vi "Configure.vi"(8 "error in (no error)":errorcluster, 11 "Tomo in":refnum<class "Tomo.lvclass">) -> (0 "error out":errorcluster, 2 "cancelled?":bool, 3 "Tomo out":refnum<class "Tomo.lvclass">)   [LabVIEW 2012, in "Tomo.lvclass"]
doc: "The configure method configures the details for the RabbitMQ connection. \n\nIn the derived class, make a call to the parent for setting these parameters."
uses:
  Tomo.lvclass
  <vilib>/Utility/miscctls.llb/LVPointTypeDef.ctl
  Tomo.lvclass/Tomo.ctl
  <vilib>/Distrio/Murmex/Murmex/Murmex.lvclass
panel:
  in  "stack overhead time":dbl[unit]
  in  "default stages speed":dbl[unit]
  in  "button::cancel":bool
  in  "button::configure_murmex":bool
  in  "button::ok":bool
  in  "mapping file folder":path
  in  "stages component":string
  in  "camera component":string
  in  "stack component":string
  # "Slave components names"
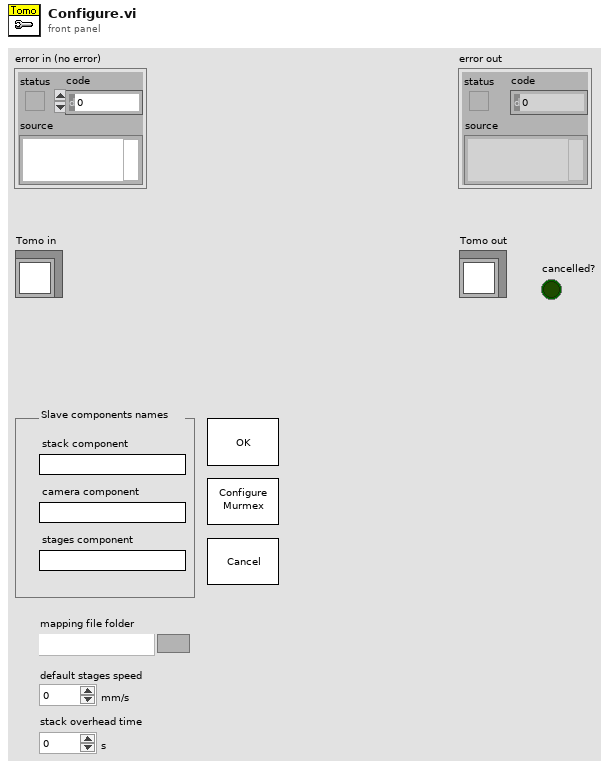
[diagram p1: front panel]
types:
  T1 = typedef "LVPointTypeDef.ctl" = cluster{"Horizontal":i16, "Vertical":i16}
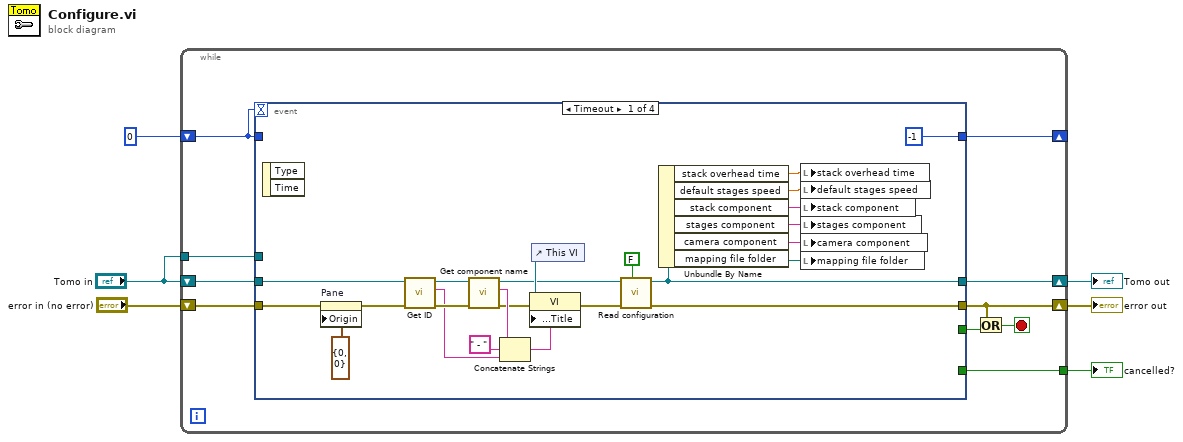
[diagram p0: block diagram]
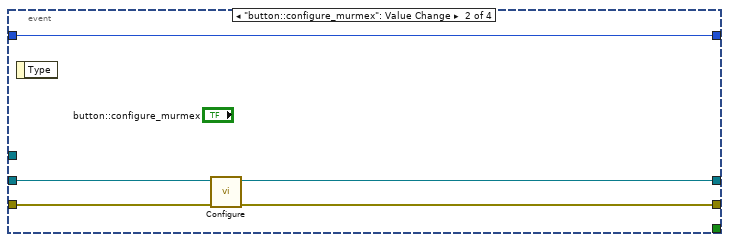
[diagram p2: hidden frame]
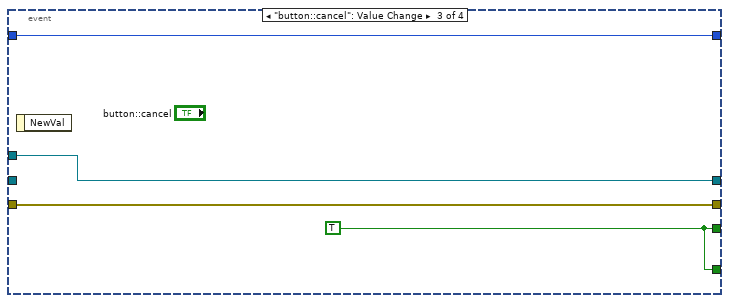
[diagram p3: hidden frame]
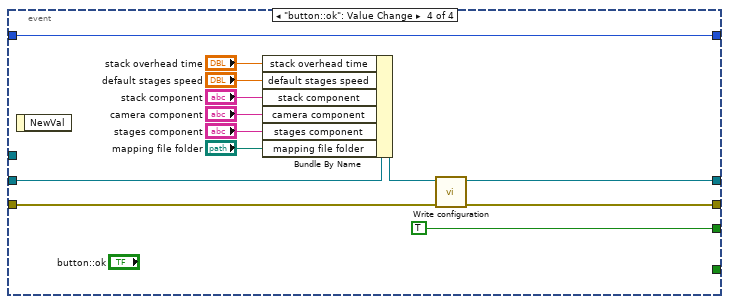
[diagram p4: hidden frame]
diagram:
  n1 = while {
    shift-right: [w9] -> w2
    shift-left: "error in (no error)" -> [w16]
    shift-right: [w12] -> _
    shift-left: 0 -> [w15]
    shift-right: [w11] -> w1
    shift-left: "Tomo in" -> [w14]
    tunnel: "Tomo in" -> [w13]
    tunnel: [w7] -> w3
    stop <- w8 stop-if-true
    n2 = event shown="[0] Timeout" {
      selector: _ -> [_ _ _ _]
      dyn-events: _ -> [_ _ _ _]
      timeout: w15 -> [_ _ _ _]
      tunnel: w16 -> [w40 w45 w48 w58]
      tunnel: w15 -> [_ w41 w46 w62]
      tunnel: w14 -> [w37 w43 _ w57]
      tunnel: w13 -> [_ _ w49 _]
      tunnel: [-1 w41 w46 w62] -> w12
      tunnel: [w23 w42 w49 w59] -> w11
      tunnel: [w24 w44 w48 w61] -> w9
      tunnel: [_ _ w47 TRUE] -> w10
      tunnel: [_ _ w47 _] -> w7
      event Timeout {
        n3 = event-data() -> ()  [unwired: 1 in, 2 out]
        n4 = property on="Pane" class="Pane"(error in=w40, "Origin"=T1 {"Horizontal"=0, "Vertical"=0}) -> (error out=w38:errorcluster)  [unwired: 1 in, 1 out]
        n5 = call <vilib>:"Get ID.vi"("error in (no error)"=w38, "Murmex in"=w37) -> ("error out"=w36:errorcluster, "component id"=w33:string, "Murmex out"=w35:refnum<class "Tomo.lvclass">)  [unwired: 7 in]
        n6 = call <vilib>:"Get component name.vi"("error in (no error)"=w36, "Murmex in"=w35) -> ("error out"=w30:errorcluster, "component name"=w34:string, "Murmex out"=w26:refnum<class "Tomo.lvclass">)  [unwired: 7 in]
        n7 = Concatenate Strings(w34, " - " ("string"), w33) -> (w28:string)
        n8 = control-ref of="This VI"() -> (w29:refnum<vi>)
        n9 = property class="VI"(reference=w29, error in=w30, "Front Panel.Title"=w28) -> (error out=w27:errorcluster)  [unwired: 1 out]
        n10 = call-dynamic "Read configuration.vi"("force loading?"=FALSE, "error in (no error)"=w27, "Tomo in"=w26) -> ("error out"=w24:errorcluster, "Tomo out"=w23:refnum<class "Tomo.lvclass">)  [unwired: 7 in]
        n11 = Unbundle By Name(w23) -> ("stack overhead time"=w18:dbl[unit], "default stages speed"=w17:dbl[unit], "stack component"=w19:string, "stages component"=w20:string, "camera component"=w21:string, "mapping file folder"=w22:path)
        n12 = local write "stack overhead time"(w18) -> ()
        n13 = local write "default stages speed"(w17) -> ()
        n14 = local write "stack component"(w19) -> ()
        n15 = local write "stages component"(w20) -> ()
        n16 = local write "camera component"(w21) -> ()
        n17 = local write "mapping file folder"(w22) -> ()
      }
      event "button::configure_murmex": Value Change {
        n18 = event-data() -> ()  [unwired: 1 in, 1 out]
        n19 = call-parent "Configure.vi"("error in (no error)"=w45, "Murmex in"=w43) -> ("error out"=w44:errorcluster, "Murmex out"=w42:refnum<class "Tomo.lvclass">)  [unwired: 7 in, 1 out]
      }
      event "button::cancel": Value Change {
        w47 = TRUE
        n20 = event-data() -> ()  [unwired: 1 in, 1 out]
      }
      event "button::ok": Value Change {
        n21 = event-data() -> ()  [unwired: 1 in, 1 out]
        n22 = Bundle By Name(cluster=w57, "stack overhead time"="stack overhead time", "default stages speed"="default stages speed", "stack component"="stack component", "camera component"="camera component", "stages component"="stages component", "mapping file folder"="mapping file folder") -> (w56:refnum<class "Tomo.lvclass">)
        n23 = call-dynamic "Write configuration.vi"("error in (no error)"=w58, "Tomo in"=w56) -> ("error out"=w61:errorcluster, "Tomo out"=w59:refnum<class "Tomo.lvclass">)  [unwired: 8 in]
      }
    }
    n24 = Or(x=w9, y=w10) -> (x .or. y?=w8:bool)
  }
  "error out" <- w2
  "Tomo out" <- w1
  "cancelled?" <- w3
